vi "TDT-Wait For Status.vi"(2 "NOT":bool, 7 "Status":i32=4 format="%x", 11 "error in (no error)":errorcluster) -> (15 "error out":errorcluster)   [LabVIEW 2020]
uses:
  TDT-Globals.vi
panel:
  out "Array":i32[](array[numeric])
  in  "Timeout (ms)":u32=5000
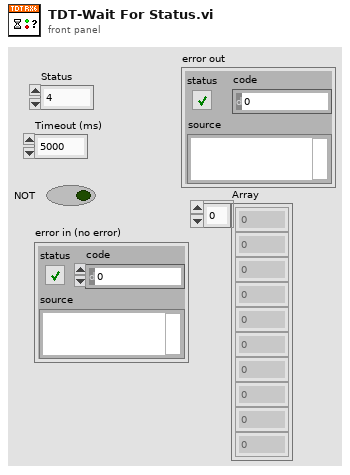
[diagram p1: front panel]
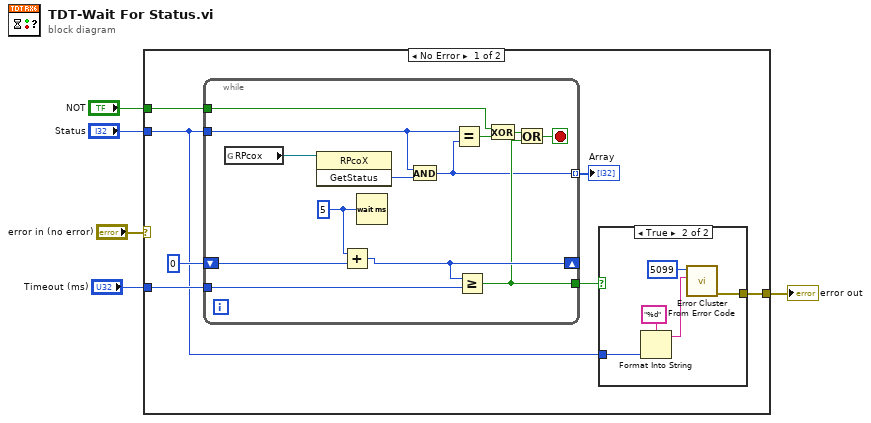
[diagram p0: block diagram]
diagram:
  n1 = case shown="No Error" "error in (no error)" {
    selector: "error in (no error)" -> [_ w31]
    tunnel: "Timeout (ms)" -> [w11 _]
    tunnel: [w9 w31] -> w4
    tunnel: "Status" -> [w8 _]
    tunnel: "NOT" -> [w6 _]
    frame No Error {
      n2 = while {
        tunnel: w8 -> [w27]
        shift-right: [w24] -> _
        shift-left: 0 -> [w26]
        tunnel: w11 -> [w23]
        tunnel: [w21] -> w10
        tunnel: w6 -> [w19]
        tunnel: [w18] -> w7 mode=indexing
        stop <- w22 stop-if-true
        w25 = u32 5 ("milliseconds to wait")
        n3 = global read "TDT-Globals.vi" "RPcox"() -> (w29:refnum<k7>)
        n4 = invoke class="RPcoX" method="GetStatus"(reference=w29) -> ("GetStatus"=w30:i32)  [unwired: 2 in, 2 out]
        n5 = Add(x=w25, y=w26) -> (x+y=w24:u32)
        n6 = Wait (ms)(milliseconds to wait=w25) -> ()  [unwired: 1 out]
        n7 = And(x=w27, y=w30) -> (x .and. y?=w18:i32)
        n8 = Equal?(x=w27, y=w18) -> (x = y?=w28:bool)
        n9 = Greater Or Equal?(x=w24, y=w23) -> (x >= y?=w21:bool)
        n10 = Exclusive Or(1:w28, 2:w19) -> (0:w20:bool)
        n11 = Or(x=w20, y=w21) -> (x .or. y?=w22:bool)
      }
      "Array" <- w7
      n12 = case shown="True" w10 {
        tunnel: [_ w16] -> w9
        tunnel: w8 -> [_ w13]
        frame False {
        }
        frame True {
          n13 = Format Into String(format string="%d", w13) -> (resulting string=w14:string)  [unwired: 2 in, 1 out]
          n14 = call <vilib>:"Error Cluster From Error Code.vi"("error message (\"\")"=w14, "error code (0)"=5099) -> ("error out"=w16:errorcluster)  [unwired: 7 in]
        }
      }
    }
    frame Error {
    }
  }
  "error out" <- w4
